vi "SSC DCPower Configure Voltage Sequence without Ramp.vi"(0 "DCPower SSC in":T1[](array[typedef]), 5 "Voltage Sequence In":dbl[](array[numeric]), 7 "Source Delays in":dbl[](array[numeric]), 11 "error in":errorcluster) -> (4 "DCPower SSC out":T1[](array[typedef]), 15 "error out":errorcluster)   [LabVIEW 2019]
doc: "This VI configures the Voltage Level in Sequence\nIt can generate volt from low to high and vice versa"
uses:
  Instrument Control/DCPower/SSC DCPower/SSC DCPower.ctl
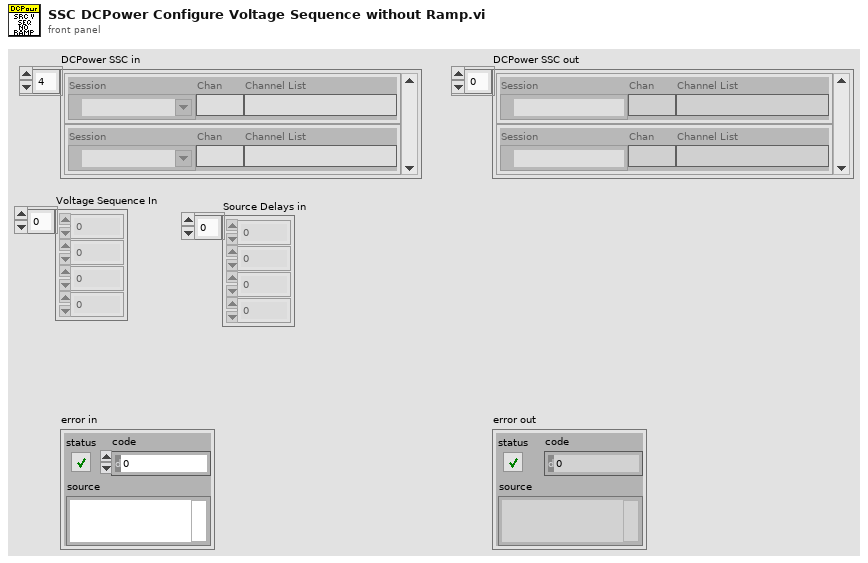
[diagram p1: front panel]
types:
  T1 = typedef "SSC DCPower.ctl" = cluster{"Session":refnum<k15>, "Chan":string, "Channel List":string}
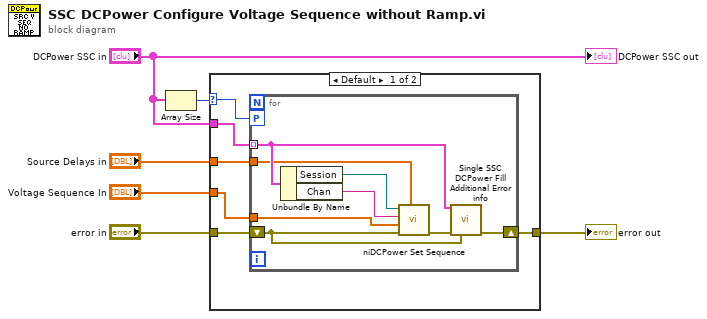
[diagram p0: block diagram]
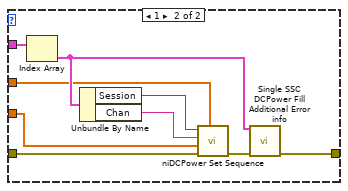
[diagram p2: hidden frame]
diagram:
  n1 = Array Size(array="DCPower SSC in") -> (size(s)=w5:i32)
  n2 = case shown="Default" w5 {
    selector: w5 -> [w10 _]
    tunnel: [w12 w29] -> w6
    tunnel: "error in" -> [w11 w28]
    tunnel: "DCPower SSC in" -> [w9 w27]
    tunnel: "Voltage Sequence In" -> [w8 w22]
    tunnel: "Source Delays in" -> [w7 w21]
    frame Default {
      n3 = for {
        tunnel: w9 -> [w17] mode=indexing
        workers-P: w10 -> [_]
        shift-right: [w18] -> w12
        shift-left: w11 -> [w14]
        tunnel: w8 -> [w16]
        tunnel: w7 -> [w13]
        n4 = Unbundle By Name(w17) -> ("Session"=w20:refnum<k15>, "Chan"=w19:string)
        n5 = call <instrlib>:"niDCPower Set Sequence.vi"("source delays"=w13, "error in (no error)"=w14, "values"=w16, "channel name"=w19, "instrument handle"=w20) -> ("error out"=w15:errorcluster)  [unwired: 5 in, 1 out]
        n6 = call "Single SSC DCPower Fill Additional Error info.vi"("DCPower SSC in"=w17, "error in"=w15, "previous error in"=w14) -> ("error out"=w18:errorcluster)  [unwired: 12 in]
      }
    }
    frame 1 {
      n7 = Index Array(array=w27) -> (element=w23:T1)  [unwired: 1 in]
      n8 = Unbundle By Name(w23) -> ("Session"=w25:refnum<k15>, "Chan"=w24:string)
      n9 = call <instrlib>:"niDCPower Set Sequence.vi"("source delays"=w21, "error in (no error)"=w28, "values"=w22, "channel name"=w24, "instrument handle"=w25) -> ("error out"=w26:errorcluster)  [unwired: 5 in, 1 out]
      n10 = call "Single SSC DCPower Fill Additional Error info.vi"("DCPower SSC in"=w23, "error in"=w26, "previous error in"=w28) -> ("error out"=w29:errorcluster)  [unwired: 12 in]
    }
  }
  "error out" <- w6
  "DCPower SSC out" <- "DCPower SSC in"
